vi "setManual.vi"(0 "Interface in":T2, 5 "PI_Controller":T1, 7 "manual":sgl format="%#_13g", 11 "error in":errorcluster) -> (4 "Interface out":T2, 15 "error out":errorcluster)   [LabVIEW 2017, in "AFE_interface.lvlib"]
uses:
  AFE_interface.lvlib
  InterfaceRef.ctl
  <instrlib>/_niInstr/Instruction Framework/v1/Host/Instruction Target/niInstr Instruction Target v1 Host.lvclass
  <instrlib>/_niInstr/Instruction Framework/v1/Host/Instruction Framework Context/niInstr Instruction Framework Context v1 Host.lvclass
  PI_Controllers.ctl
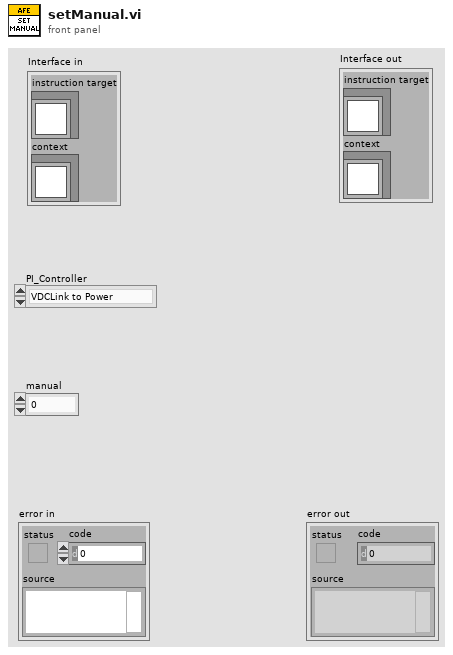
[diagram p1: front panel]
types:
  T1 = typedef "AFE_interface.lvlib/PI_Controllers.ctl" = enum16{"VDCLink to Power", "ID to VD", "IQ to VQ"}
  T2 = typedef "AFE_interface.lvlib/InterfaceRef.ctl" = cluster{"instruction target":refnum<class "niInstr Instruction Target v1 Host.lvclass">, "context":refnum<class "niInstr Instruction Framework Context v1 Host.lvclass">}
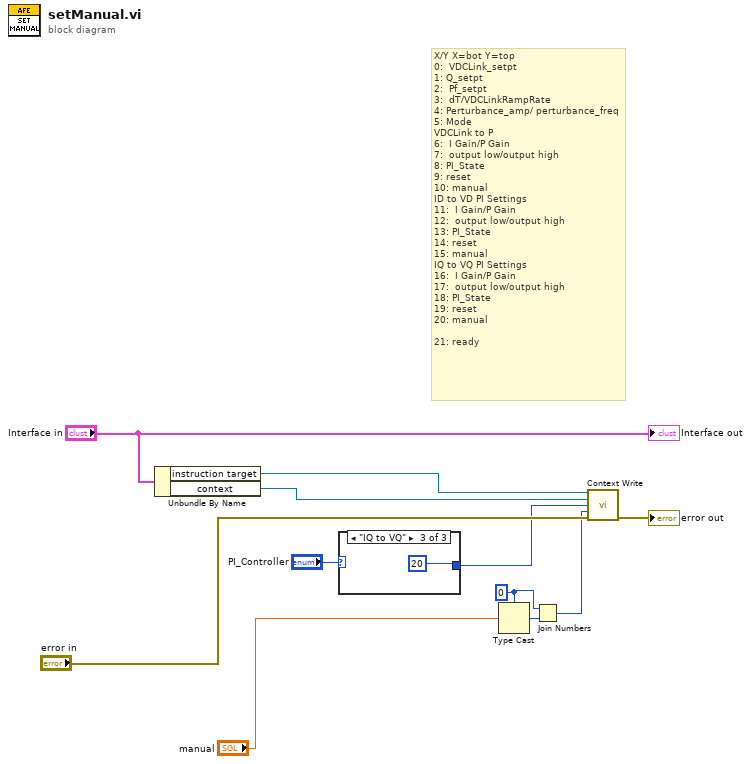
[diagram p0: block diagram]
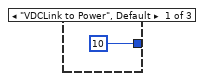
[diagram p2: hidden frame]
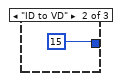
[diagram p3: hidden frame]
diagram:
  w6 = u32 0
  # "X/Y X=bot Y=top\n0:  VDCLink_setpt\n1: Q_setpt\n2:  Pf_setpt\n3:  dT/VDCLinkRampRate\n4: Perturbance_amp/ perturbance_freq\n5: Mode\nVDCLink to P\n6:  I Gain/P Gain\n7:  output low/output high\n8: PI_State\n9: reset\n10: manual\nID to VD PI Settings \n11:  I Gain/P Gain\n12:  output low/output high\n13: PI_State\n14: reset\n15: manual\nIQ to VQ PI Settings\n16:  I Gain/P Gain\n17:  output low/output high\n18: PI_State\n19: reset\n20: manual\n\n21: ready"
  n1 = Unbundle By Name("Interface in") -> ("instruction target"=w10:refnum<class "niInstr Instruction Target v1 Host.lvclass">, "context"=w9:refnum<class "niInstr Instruction Framework Context v1 Host.lvclass">)
  n2 = case shown="\"IQ to VQ\"" "PI_Controller" {
    tunnel: [u64 10 ("address") u64 15 ("address") u64 20 ("address")] -> w1
    frame "VDCLink to Power", Default {
    }
    frame "ID to VD" {
    }
    frame "IQ to VQ" {
    }
  }
  n3 = Type Cast(type=w6, x="manual") -> (*(type *) &x=w7:u32)
  n4 = Join Numbers(hi=w6, lo=w7) -> ((hi.lo)=w3:u64)
  n5 = call <instrlib>:"Context Write.vi"("instruction target in"=w10, "context in"=w9, "address"=w1, "data"=w3, "error in"="error in") -> ("error out"=→"error out":errorcluster)  [unwired: 8 in, 2 out]
  "Interface out" <- "Interface in"
